vi "ep_Append 2D Array.vi"(9 "samples per cycle":u16=192, 10 "current data":dbl[][](array[numeric]), 11 "history data":dbl[][](array[numeric])) -> (1 "total size":i32, 2 "total cycles":i32, 3 "appended data":dbl[][](array[numeric]))   [LabVIEW 2013, in "NI_EP_Power Measurement.lvlib"]
uses:
  <vilib>/addons/Electrical Power/Power Measurement/NI_EP_Power Measurement.lvlib
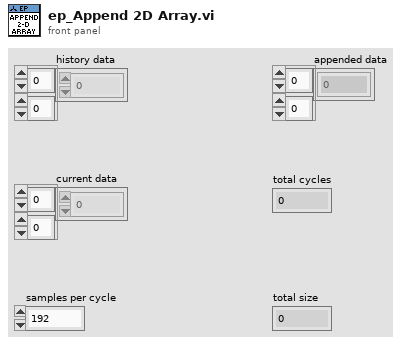
[diagram p1: front panel]
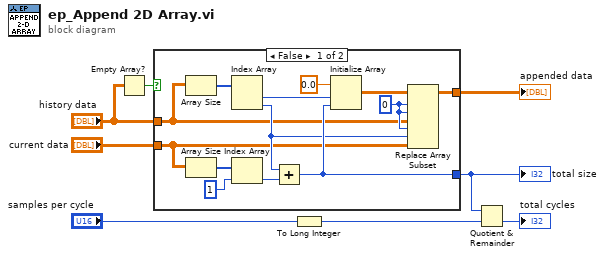
[diagram p0: block diagram]
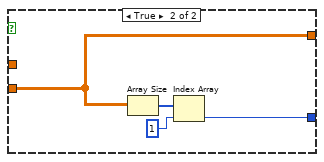
[diagram p2: hidden frame]
diagram:
  n1 = Empty Array?(array="history data") -> (empty?=w5:bool)
  n2 = case shown="False" w5 {
    tunnel: "current data" -> [w10 w23]
    tunnel: [w14 w23] -> w8
    tunnel: "history data" -> [w11 _]
    tunnel: [w13 w22] -> w1
    frame False {
      w16 = 0 ("index (row)")
      n3 = Array Size(array=w11) -> (size(s)=w21:i32[])
      n4 = Array Size(array=w10) -> (size(s)=w20:i32[])
      n5 = Index Array(array=w21) -> (element #1=w9:i32, element #2=w12:i32)  [unwired: 2 in]
      n6 = Index Array(array=w20, index=1) -> (element=w15:i32)
      n7 = Add(x=w12, y=w15) -> (x+y=w13:i32)
      n8 = Initialize Array(0.0 ("element"), w9, w13) -> (w17:dbl[][])
      n9 = Replace Array Subset(array=w17, new element #1=w11, index (row) #1=w16, index (col) #1=w16, new element #2=w10, index (row) #2=w16, index (col) #2=w12) -> (w14:dbl[][])
    }
    frame True {
      n10 = Array Size(array=w23) -> (size(s)=w24:i32[])
      n11 = Index Array(array=w24, index=1) -> (element=w22:i32)
    }
  }
  "appended data" <- w8
  "total size" <- w1
  n12 = To Long Integer(number="samples per cycle") -> (32bit integer=w3:i32)
  n13 = Quotient & Remainder(x=w1, y=w3) -> (floor(x/y)=→"total cycles":i32)  [unwired: 1 out]
